vi "Measurement A.vi"(0 "Inputs":T1, 7 "First name":string, 9 "Last name":string) -> (4 "Result":dbl, 8 "Full name":string)   [LabVIEW 2021]
uses:
  controls/Measurement Inputs.ctl
  controls/Offset value.ctl
  Reusables/controls/Username.ctl
  Meas A.lvlib
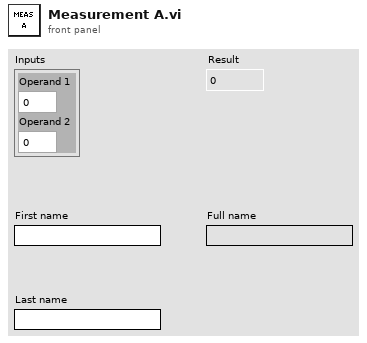
[diagram p1: front panel]
types:
  T1 = typedef "Meas A.lvlib/Measurement Inputs.ctl" = cluster{"Operand 1":dbl, "Operand 2":dbl}
  T2 = typedef "Username.ctl" = cluster{"First name":string, "Last name":string}
  T3 = typedef "Meas A.lvlib/Offset value.ctl" = cluster{"offset":dbl}
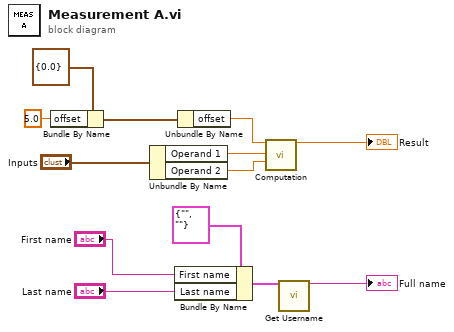
[diagram p0: block diagram]
diagram:
  n1 = Bundle By Name(cluster=T3 {"offset"=0.0}, "offset"=5.0) -> (w6:T3)
  n2 = Unbundle By Name("Inputs") -> ("Operand 1"=w12:dbl, "Operand 2"=w11:dbl)
  n3 = Bundle By Name(cluster=T2 {"First name"="", "Last name"=""} ("Name"), "First name"="First name", "Last name"="Last name") -> (w4:T2)
  n4 = Unbundle By Name(w6) -> ("offset"=w10:dbl)
  n5 = call "Computation.vi"("offset"=w10, "Operand 1"=w12, "Operand 2"=w11) -> ("Result"=→"Result":dbl)  [unwired: 12 in]
  n6 = call "Get Username.vi"("Name"=w4) -> ("Full name"=→"Full name":string)  [unwired: 14 in]
